vi "Acquire Data from Hardware.vi"(7 "error in (no error)":errorcluster caption="错误输入（无错误）", 10 "Hardware Configuration":T1 caption="硬件配置") -> (0 "error out":errorcluster caption="错误输出", 2 "Graph Data":waveform(dbl)[](array[waveform]) caption="图形数据")   [LabVIEW 2013]
doc: "按硬件配置输入中的信号类型，生成采样波形。"
uses:
  controls/HW Configuration.ctl
  <vilib>/DAQmx/read.llb/DAQmx Read (Analog 1D Wfm NChan NSamp).vi
  <vilib>/DAQmx/create/channels.llb/DAQmx Create Channel (AI-Voltage-Basic).vi
  <vilib>/DAQmx/configure/timing.llb/DAQmx Timing (Sample Clock).vi
  <vilib>/DAQmx/miscellaneous.llb/DAQmx Fill In Error Info.vi
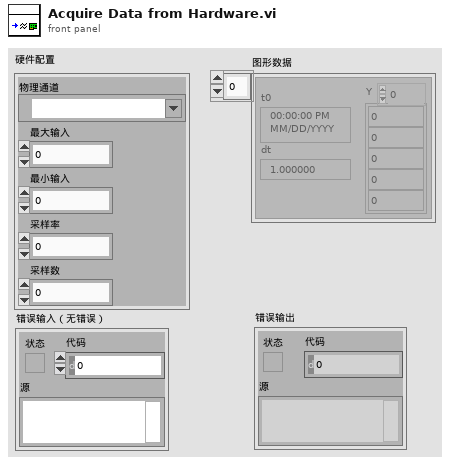
[diagram p1: front panel]
types:
  T1 = typedef "HW Configuration.ctl" = cluster{"Physical Channel":tag, "Maximum Input":dbl, "Minimum Input":dbl, "Sample Rate":dbl, "Number of Samples":i32}
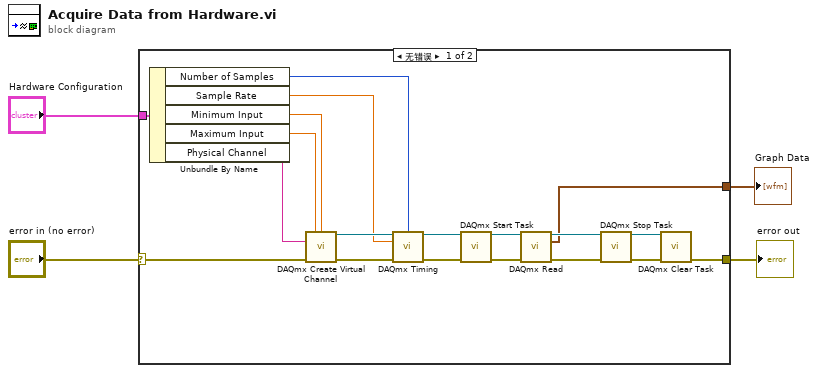
[diagram p0: block diagram]
diagram:
  n1 = case shown="无错误" "error in (no error)" {
    selector: "error in (no error)" -> [w14 w24]
    tunnel: [w15 w24] -> w3
    tunnel: "Hardware Configuration" -> [w23 _]
    tunnel: [w18 _] -> w1
    frame No Error {
      n2 = Unbundle By Name(w23) -> ("Number of Samples"=w7:i32, "Sample Rate"=w8:dbl, "Minimum Input"=w11:dbl, "Maximum Input"=w12:dbl, "Physical Channel"=w13:tag)
      n3 = call-poly <vilib>:"DAQmx Create Virtual Channel.vi"("maximum value"=w12, "minimum value"=w11, "physical channels"=w13, "error in"=w14) -> ("task out"=w9:refnum<k21>, "error out"=w10:errorcluster)  [unwired: 10 in]
      n4 = call-poly <vilib>:"DAQmx Timing.vi"("task/channels in"=w9, "samples per channel"=w7, "rate"=w8, "error in"=w10) -> ("task out"=w6:refnum<k21>, "error out"=w5:errorcluster)  [unwired: 10 in]
      n5 = call <vilib>:"DAQmx Start Task.vi"("task/channels in"=w6, "error in"=w5) -> ("task out"=w22:refnum<k21>, "error out"=w21:errorcluster)  [unwired: 12 in]
      n6 = call-poly <vilib>:"DAQmx Read.vi"("task/channels in"=w22, "error in"=w21) -> ("task out"=w19:refnum<k21>, "data"=w18:waveform(dbl)[], "error out"=w20:errorcluster)  [unwired: 11 in]
      n7 = call <vilib>:"DAQmx Stop Task.vi"("task/channels in"=w19, "error in"=w20) -> ("task out"=w16:refnum<k21>, "error out"=w17:errorcluster)  [unwired: 12 in]
      n8 = call <vilib>:"DAQmx Clear Task.vi"("task in"=w16, "error in"=w17) -> ("error out"=w15:errorcluster)  [unwired: 13 in]
    }
    frame Error {
    }
  }
  "error out" <- w3
  "Graph Data" <- w1
